vi "Histogram0007.vi"   [LabVIEW 2013]
uses:
  <vilib>/Heliosphere Research LLC/Advanced Plotting Toolkit/api_core/NewPlotScales.ctl
  <vilib>/Heliosphere Research LLC/Advanced Plotting Toolkit/api_plotting/Histogram_Automatic.vi
  <vilib>/Heliosphere Research LLC/Advanced Plotting Toolkit/Advanced Plotting Toolkit.lvlib
types:
  T1 = typedef "Advanced Plotting Toolkit.lvlib/NewPlotScales.ctl" = enum16{"Default", "Linear", "Log", "Symlog"}
  T2 = typedef "Advanced Plotting Toolkit.lvlib/PlotID.ctl" = i32
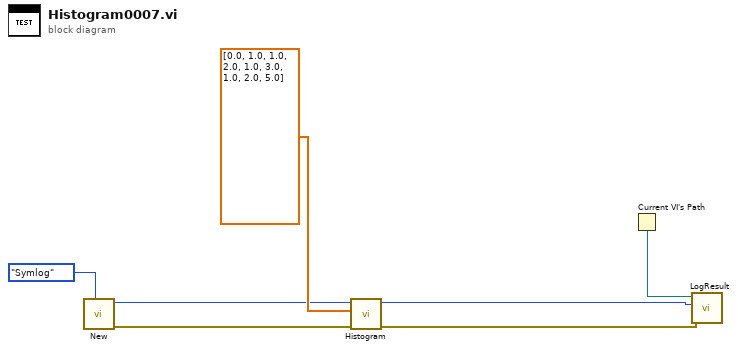
[diagram p0: block diagram]
diagram:
  n1 = call <vilib>:"New.vi"("X Axis Scale"=NewPlotScales."Symlog") -> ("error out"=w1:errorcluster, "Plot ID"=w2:T2)  [unwired: 9 in]
  n2 = call-poly <vilib>:"Histogram.vi"("error in (no error)"=w1, "Data"=dbl[] [0.0, 1.0, 1.0, 2.0, 1.0, 3.0, 1.0, 2.0, 5.0], "Plot ID"=w2) -> ("error out"=w5:errorcluster, "Plot ID Out"=w7:T2)  [unwired: 7 in]
  n3 = Current VI's Path() -> (path=w6:path)
  n4 = call "LogResult.vi"("Test Result"=w5, "Test Artifact"=w7, "VI Path"=w6) -> ()  [unwired: 9 in]
